vi "GetType.vi"(8 "error in (no error)":errorcluster, 11 "Write Single Calibration Curve to Instrument Msg":refnum<class "Write Single Calibration Curve to Instrument Msg.lvclass">) -> (0 "error out":errorcluster, 2 "Data Sample":variant, 3 "Write Single Calibration Curve to Instrument Msg":refnum<class "Write Single Calibration Curve to Instrument Msg.lvclass">)   [LabVIEW 2016, in "LS218.lvlib" / "Write Single Calibration Curve to Instrument Msg.lvclass"]
uses:
  Write Single Calibration Curve to Instrument Msg.lvclass
  Write Single Calibration Curve to Instrument Msg.lvclass/Write Single Calibration Curve to Instrument Msg.ctl
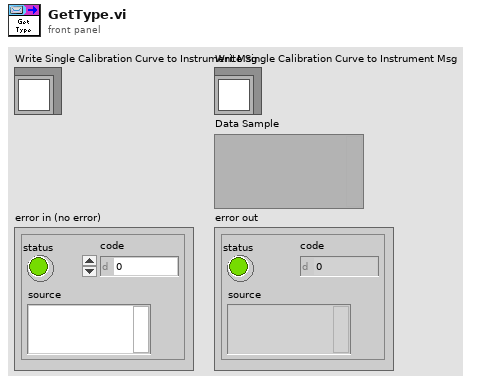
[diagram p1: front panel]
types:
  T1 = cluster{"Calibration File":path, "Channel":i32, "Sensor Type":u16, "Display Source":u16}
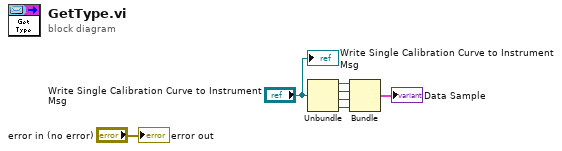
[diagram p0: block diagram]
diagram:
  n1 = Unbundle("Write Single Calibration Curve to Instrument Msg") -> (w4:path, w3:i32, w2:u16, w1:u16)
  n2 = Bundle("Calibration File"=w4, "Channel"=w3, "Sensor Type"=w2, "Display Source"=w1) -> (→"Data Sample":T1)  [unwired: 1 in]
  "error out" <- "error in (no error)"
  "Write Single Calibration Curve to Instrument Msg" <- "Write Single Calibration Curve to Instrument Msg"
